vi "MathCad_String_Set.vi"(0 "Worksheet Reference In":refnum<k7>, 2 "value":string, 5 "Mathcad.IStringValue":refnum<k7>, 11 "error in":errorcluster) -> (4 "Worksheet Reference Out":refnum<k7>, 6 "Mathcad.IStringValue Out":refnum<k7>, 15 "error out":errorcluster)   [LabVIEW 2015]
doc: "Sets the value of the reference. This must be done before inserting into a worksheet."
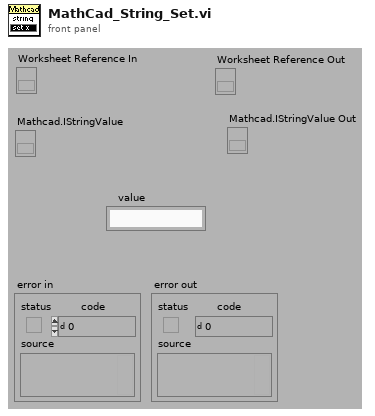
[diagram p1: front panel]
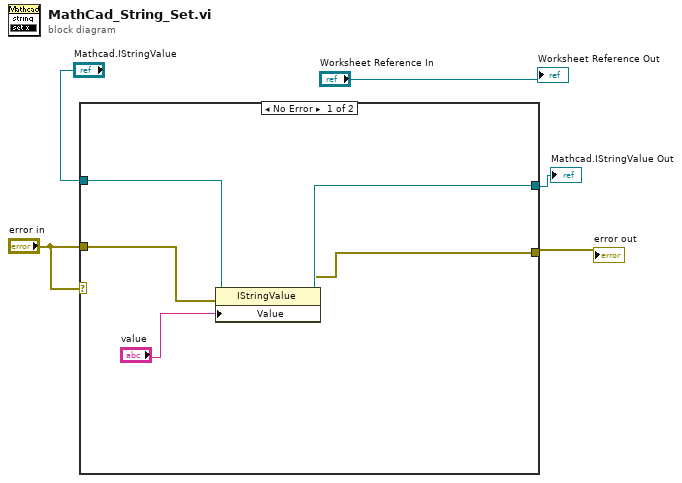
[diagram p0: block diagram]
diagram:
  n1 = case shown="No Error" "error in" {
    tunnel: "error in" -> [w9 w12]
    tunnel: [w8 w12] -> w5
    tunnel: "Mathcad.IStringValue" -> [w7 w11]
    tunnel: [w10 w11] -> w1
    frame No Error {
      n2 = property class="IStringValue"(reference=w7, error in=w9, "Value"="value") -> (reference out=w10:refnum<k7>, error out=w8:errorcluster)
    }
    frame Error {
    }
  }
  "error out" <- w5
  "Mathcad.IStringValue Out" <- w1
  "Worksheet Reference Out" <- "Worksheet Reference In"
